vi "Settings1.vi"(9 "Numeric Control":dbl, 10 "Value":dbl, 11 "Enable":bool) -> (3 "Numeric Indicator":dbl)   [LabVIEW 2011]
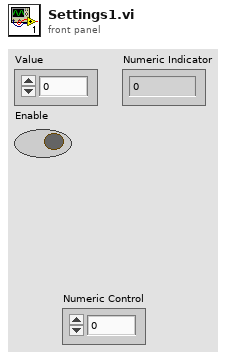
[diagram p1: front panel]
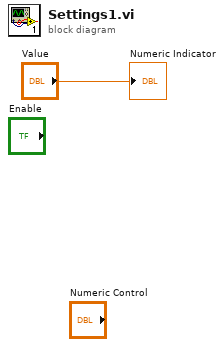
[diagram p0: block diagram]
diagram:
  "Numeric Indicator" <- "Value"
